vi "Increment Counter.vi"(7 "Method Name":string, 10 "Status":T1=enum."Passed", 11 "Test Result Tree V2 in":refnum<class "Test Result Tree V2.lvclass">) -> (3 "Test Result Tree V2 out":refnum<class "Test Result Tree V2.lvclass">)   [LabVIEW 2020, in "Test Result Tree V2.lvclass"]
uses:
  Test Result Tree V2.lvclass
  Result/Status.ctl
  Test Result Tree Test/Private/Counter Map Key.ctl
  Test Result Tree V2.lvclass/Test Result Tree V2.ctl
  <vilib>/Utility/miscctls.llb/LVMapReplaceAction.ctl
  Result/Result.lvlib
  Utilities/LUnit Utilities.lvlib
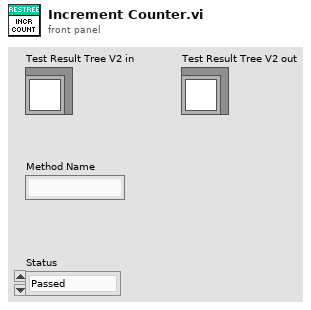
[diagram p1: front panel]
types:
  T1 = typedef "Result.lvlib/Status.ctl" = enum16{"", "Passed", "Failed", "Error", "Skipped", "Setup Error", "Broken", "Teardown Error"}
  T2 = typedef "Test Result Tree V2.lvclass/Counter Map Key.ctl" = cluster{"Test Case":string, "Status":T1}
  T3 = typedef "LVMapReplaceAction.ctl" = enum32{"Modify Entry only if found", "Add or Modify Entry", "Delete Entry"}
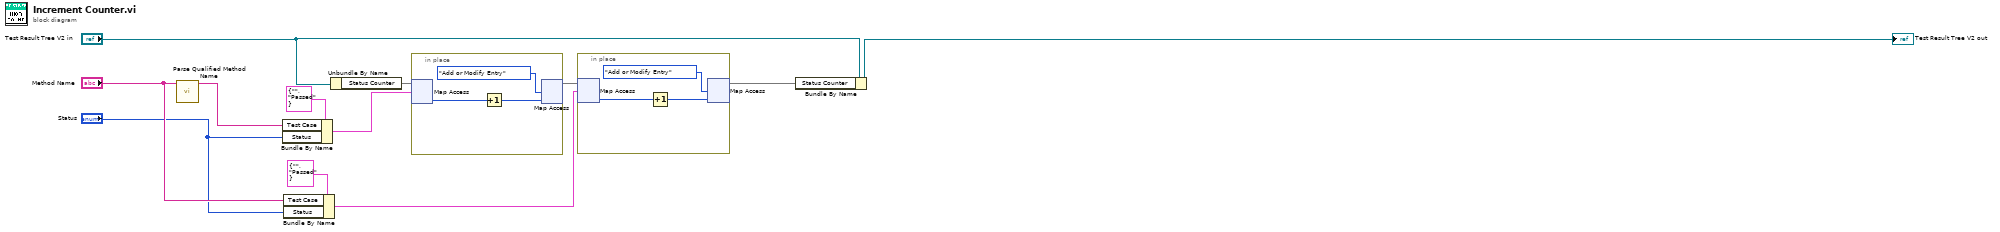
[diagram p0: block diagram]
diagram:
  n1 = call "Parse Qualified Method Name.vi"("Case"="Method Name") -> ("Test Case Class Name"=w11:string)  [unwired: 9 in, 1 out]
  n2 = Bundle By Name(cluster=T2 {"Test Case"="", "Status"=enum."Passed"} ("key"), "Test Case"=w11, "Status"="Status") -> (w10:T2)
  n3 = Bundle By Name(cluster=T2 {"Test Case"="", "Status"=enum."Passed"} ("key"), "Test Case"="Method Name", "Status"="Status") -> (w1:T2)
  n4 = Unbundle By Name("Test Result Tree V2 in") -> ("Status Counter"=w7:map{T2, i32})
  n5 = in-place {
    n6 = in-place-map #1(w7, w10) -> (w15:i32)  [unwired: 1 in, 1 out]
    n7 = Increment(x=w15) -> (x+1=w14:i32)
    n8 = in-place-map #1(w14, LVMapReplaceAction."Add or Modify Entry" ("action")) -> (w3:map{T2, i32})  [unwired: 2 out]
  }
  n9 = in-place {
    n10 = in-place-map #2(w3, w1) -> (w18:i32)  [unwired: 1 in, 1 out]
    n11 = Increment(x=w18) -> (x+1=w17:i32)
    n12 = in-place-map #2(w17, LVMapReplaceAction."Add or Modify Entry" ("action")) -> (w2:map{T2, i32})  [unwired: 2 out]
  }
  n13 = Bundle By Name(cluster="Test Result Tree V2 in", "Status Counter"=w2) -> (→"Test Result Tree V2 out":refnum<class "Test Result Tree V2.lvclass">)
